vi "Read state control indices.vi"(11 "user tag bus module in":refnum<class "user tag bus module.lvclass">) -> (2 "state control":T1, 3 "user tag bus module out":refnum<class "user tag bus module.lvclass">)   [LabVIEW 2013, in "user tag bus module.lvclass"]
doc: "This function is intended to enable easier testing. Tests can get the indices of data without having to perform the lookup a second time."
uses:
  user tag bus module.lvclass
  state control.ctl
  user tag bus module.lvclass/user tag bus module.ctl
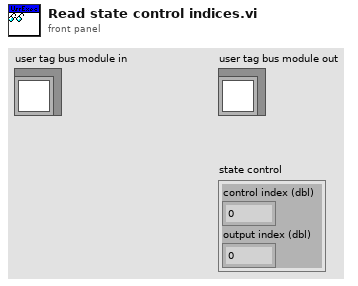
[diagram p1: front panel]
types:
  T1 = typedef "user tag bus module.lvclass/state control.ctl" = cluster{"control index (dbl)":i32, "output index (dbl)":i32}
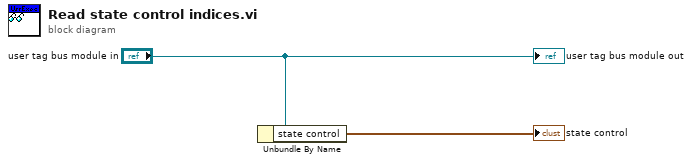
[diagram p0: block diagram]
diagram:
  n1 = Unbundle By Name("user tag bus module in") -> ("state control"=→"state control":T1)
  "user tag bus module out" <- "user tag bus module in"
